vi "teste_sobe_rampa.vi"() -> ()   [LabVIEW 2016]
uses:
  <vilib>/NXT/Subs/LVHSConnector.ctl
  <vilib>/NXT/LegoClasses/BrickReference/BrickReference.lvclass
  <vilib>/NXT/Block Support/NXT_OutputPort.ctl
  <vilib>/NXT/NXTIO Xnodes/NXTIONodeSubVIs/NXTMoveMotors.vi
  <vilib>/NXT/Dual Mode Library/Waits/Wait_Num.vi
  <vilib>/NXT/NXTIO Xnodes/NXTIONodeSubVIs/NXTStopMotors.vi
  <vilib>/NXT/NXTIO Xnodes/AddressXNode/NXTIOAddress.xnode
  <vilib>/NXT/NXTIO Xnodes/NXTIOXNode/NXTIO.xnode
panel:
  in  "NXT/EV3":T1
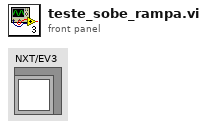
[diagram p1: front panel]
types:
  T1 = typedef "LVHSConnector.ctl" = refnum<class "BrickReference.lvclass">
  T2 = typedef "NXT_OutputPort.ctl" = u8
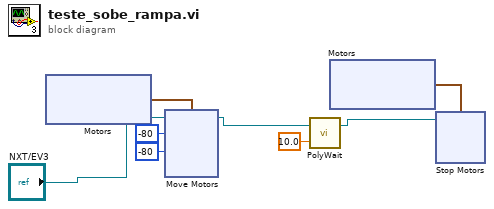
[diagram p0: block diagram]
diagram:
  n1 = xnode "Motors"() -> ("Motor"=w6:cluster{"Port":T2, "Port":T2})
  n2 = xnode "Move Motors"("Power/Speed 2"=i8 -80, "Power/Speed 1"=i8 -80, "Motors"=w6, "NXT/EV3"="NXT/EV3") -> ("NXT/EV3"=w5:T1)
  n3 = call-poly <vilib>:"PolyWait.vi"("Time (1 sec)"=sgl 10.0, "NXT/EV3"=w5) -> ("NXT/EV3"=w3:T1)  [unwired: 2 in]
  n4 = xnode "Motors"() -> ("Motor"=w2:cluster{"Port":T2, "Port":T2})
  n5 = xnode "Stop Motors"("Motors"=w2, "NXT/EV3"=w3) -> ()  [unwired: 1 out]
